vi "DMM Configuration - Update DMM Controls Items.vi"(6 "Measurement In":u16, 7 "Resolution in Digits Saved Value":dbl, 8 "error in (no error)":errorcluster, 9 "Range Ref":refnum<vi>, 10 "Resoultion in Digits Ref":refnum<vi>, 11 "Measurements Ref":refnum<vi>) -> (0 "error out":errorcluster, 1 "Resolution in Digits Array Out":dbl[](array[numeric]), 2 "Resolution in Digits Index":i32)   [LabVIEW 2015, in "DMM-SWITCH-ScanList System Explorer.lvlib"]
doc: "Measurements, Range and Resolution in Digits original type definitions from the DMM driver were very old controls. In order to use System Controls to match our Custom Device guidelines this VI was necessary to populate the new System Controls with the data from the original Type Definitions."
uses:
  DMM-SWITCH-ScanList System Explorer.lvlib
  <instrlib>/niDMM/nidmm.llb/niDMM Resolution in Digits.ctl
  Configuration Controls/DMM Config Function.ctl
panel:
  in  "Measurement Type Def":T1 caption="Function"
  in  "Resolution in Digits Type Def":T2=6.5 caption="Resolution In Digits Type Def" items=["3 1/2"=3.5, "4 1/2"=4.5, "5 1/2"=5.5, "6 1/2"=6.5, "7 1/2"=7.5]
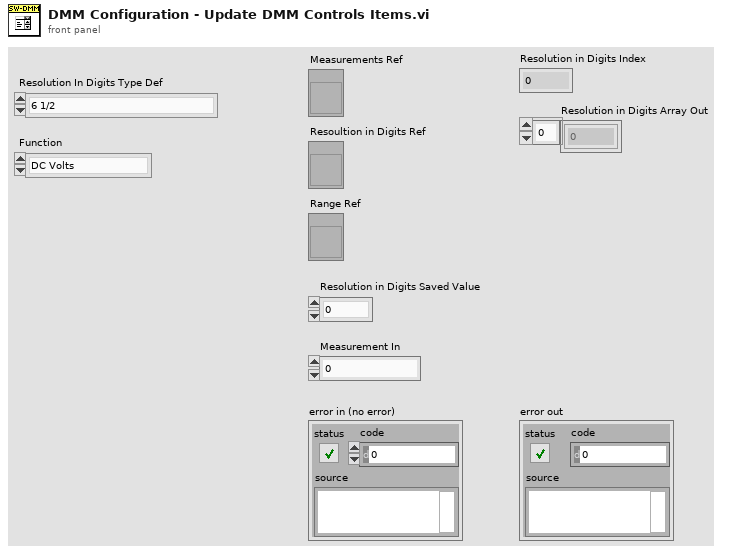
[diagram p1: front panel]
types:
  T1 = typedef "DMM-SWITCH-ScanList System Explorer.lvlib/DMM Config Function.ctl" = enum16{"DC Volts", "AC Volts", "DC Current", "AC Current", "2-wire Resistance", "4-wire Resistance", "Diode", "Frequency", "AC Volts DC Coupled", "Capacitance", "Inductance"}
  T2 = typedef "niDMM Resolution in Digits.ctl" = dbl
  T3 = typedef "LVStringsAndValuesArrayTypeDef_DBL.ctl" = cluster{"String":string, "Value":dbl}[]
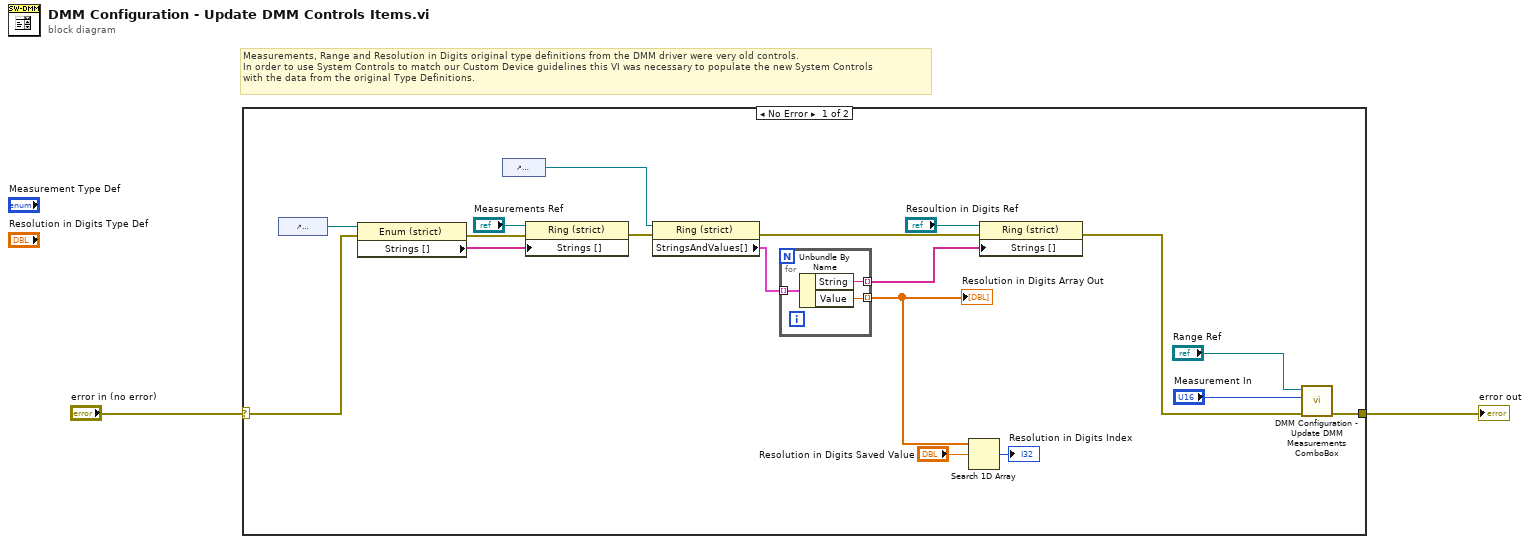
[diagram p0: block diagram]
diagram:
  # "Measurements, Range and Resolution in Digits original type definitions from the DMM driver were very old controls.\nIn order to use System Controls to match our Custom Device guidelines this VI was necessary to populate the new System Controls\nwith the data from the original Type Definitions."
  n1 = case shown="No Error" "error in (no error)" {
    selector: "error in (no error)" -> [w7 w24]
    tunnel: [w4 w24] -> w2
    frame No Error {
      n2 = control-ref of="Measurements Type Def"() -> (w9:refnum<vi>)
      n3 = property on="Property Node" class="Enum (strict)"(reference=w9, error in=w7) -> (error out=w19:errorcluster, "Strings []"=w20:string[])  [unwired: 1 out]
      n4 = control-ref of="Resolution in Digits Type Def"() -> (w8:refnum<vi>)
      n5 = property on="Property Node" class="Ring (strict)"(reference="Measurements Ref", error in=w19, "Strings []"=w20) -> (error out=w16:errorcluster)  [unwired: 1 out]
      n6 = property on="Property Node" class="Ring (strict)"(reference=w8, error in=w16) -> (error out=w18:errorcluster, "StringsAndValues[]"=w17:T3)  [unwired: 1 out]
      n7 = for {
        tunnel: w17 -> [w23] mode=indexing
        tunnel: [w22] -> w15 mode=indexing
        tunnel: [w21] -> w11 mode=indexing
        n8 = Unbundle By Name(w23) -> ("String"=w22:string, "Value"=w21:dbl)
      }
      "Resolution in Digits Array Out" <- w11
      n9 = Search 1D Array(1D array=w11, element="Resolution in Digits Saved Value") -> (index of element=→"Resolution in Digits Index":i32)  [unwired: 1 in]
      n10 = property on="Property Node" class="Ring (strict)"(reference="Resoultion in Digits Ref", error in=w18, "Strings []"=w15) -> (error out=w5:errorcluster)  [unwired: 1 out]
      n11 = call "DMM Configuration - Update DMM Measurements ComboBox.vi"("error in (no error)"=w5, "Measurement"="Measurement In", "Ring in"="Range Ref") -> ("error out"=w4:errorcluster)  [unwired: 8 in]
    }
    frame Error {
    }
  }
  "error out" <- w2
